vi "Intake Rotation Execute.vi"() -> ()   [LabVIEW 2017]
uses:
  Intake Rotation Control Type.ctl
  <vilib>/Rock Robotics/WPI/DriverStation/WPI_DriverStationRobotMode2.ctl
  Intake Rotation Notifier.ctl
  Arm Enum States.ctl
  <vilib>/Rock Robotics/WPI/ThirdParty/Phoenix-LabVIEW/Motor Controller/Controls/CTRE_Phoenix_MotorControl_ControlMode.ctl
  Intake Rotation Globals.vi
  Utility VIs/Refnum Names.vi
  Robot Global Data.vi
  Lift/Lift Globals.vi
panel:
  out "error out 3":errorcluster
  out "error out 2":errorcluster
  in  "Up kP Stow":dbl=0.001
  out "Maintain Position 2":i32
  in  "Min Output":dbl=-0.5
  in  "Max Ouput":dbl=0.6
  out "error out":errorcluster
  out "Maintain Position":i32
  in  "Lift Point":i32=6000
  in  "Kp Up":dbl=0.0003
  in  "Kp Down":dbl=0.0003
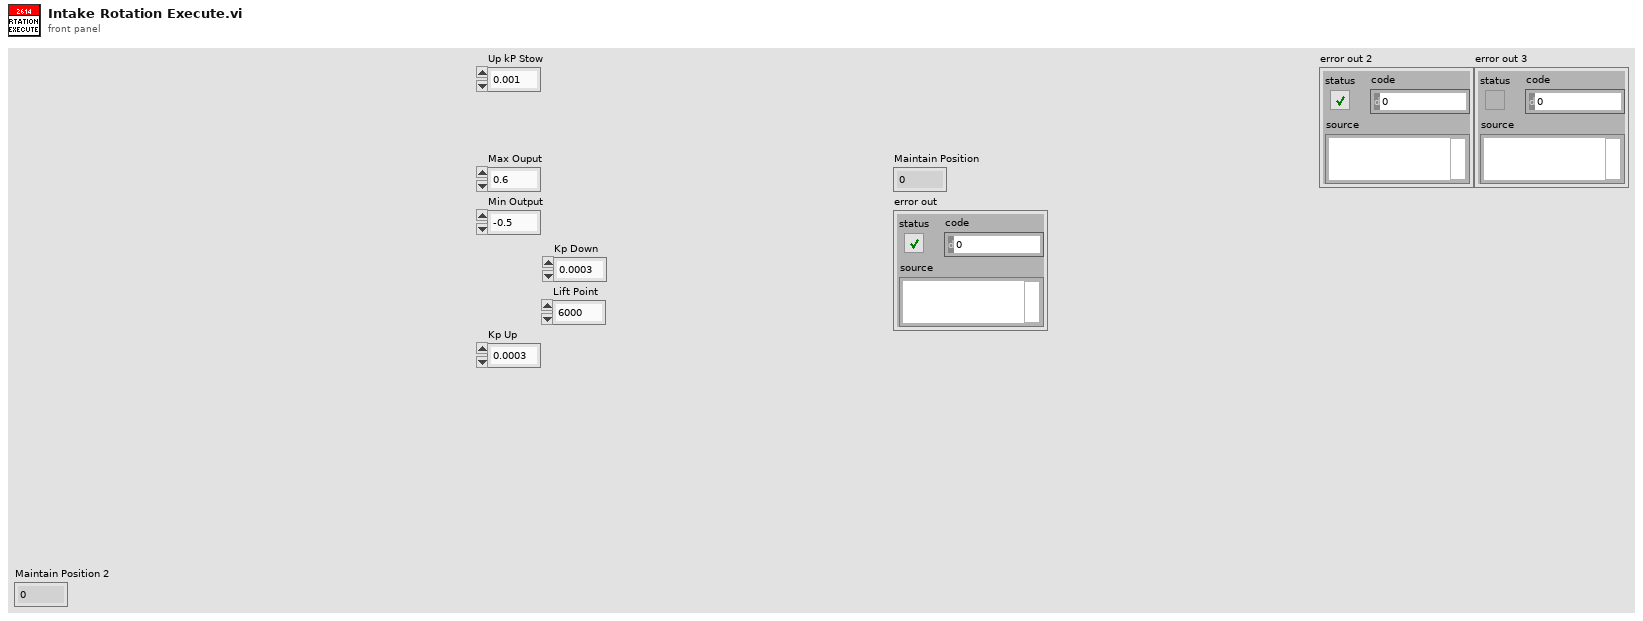
[diagram p1: front panel]
types:
  T1 = typedef "WPI_MotorControlDeviceRef.ctl" = cluster{"DeviceStatus":errorcluster, "Type":T2, "PWM":cluster{"PWM Channel":T3, "DeadBand":T4}, "CAN":cluster{"Device Number":u8, "SetOutput VI Ref":variant, "GetOutput VI Ref":variant, "Enable VI Ref":variant, "Disable VI Ref":variant, "Data":variant}, "Invert":bool, "DIO PWM":cluster{"PWM \"Enable\" Channel":T3, "DIOChannel":T5, "PWM Rate":dbl}}
  T2 = typedef "WPI_MotorControlType.ctl" = enum16{"PWM", "CAN", "DIO PWM"}
  T3 = typedef "FPGA_DIOPWMChannel.ctl" = enum8{"PWM 0", "PWM 1", "PWM 2", "PWM 3", "PWM 4", "PWM 5", "PWM 6", "PWM 7", "PWM 8", "PWM 9", "PWM MXP 0", "PWM MXP 1", "PWM MXP 2", "PWM MXP 3", "PWM MXP 4", "PWM MXP 5", "PWM MXP 6", "PWM MXP 7", "PWM MXP 8", "PWM MXP 9", "Invalid"}
  T4 = typedef "WPI_PWMDeadband.ctl" = cluster{"Name":string, "maxPositivePwm":i32, "minPositivePwm":i32, "centerPwm":i32, "maxNegativePwm":i32, "minNegativePwm":i32, "angularRange":u16}
  T5 = typedef "FPGA_DIOChannel.ctl" = enum8{"DIO 0", "DIO 1", "DIO 2", "DIO 3", "DIO 4", "DIO 5", "DIO 6", "DIO 7", "DIO 8", "DIO 9", "DIO MXP 0", "DIO MXP 1", "DIO MXP 2", "DIO MXP 3", "DIO MXP 4", "DIO MXP 5", "DIO MXP 6", "DIO MXP 7", "DIO MXP 8", "DIO MXP 9", "DIO MXP 10", "DIO MXP 11", "DIO MXP 12", "DIO MXP 13", "DIO MXP 14", "DIO MXP 15", "SPI Port CS1", "SPI Port CS2", "SPI Port CS3", "SPI Port MISO", "SPI Port MOSI", "Invalid"}
  T6 = typedef "Intake Rotation Control Type.ctl" = enum16{"No Op", "Manual Up", "Position", "Manual Down", "PositionAuto"}
  T7 = typedef "WPI_DriverStationRobotMode2.ctl" = enum16{"Autonomous Disabled", "Autonomous Enabled", "Teleop Disabled", "Teleop Enabled", "Disconnected", "Finish", "Test Disabled", "Test Enabled", "Emergency Stopped"}
  T8 = typedef "Intake Rotation Notifier.ctl" = cluster{"Step":i32, "Intake Rotation Control Type":T6, "Parameter 1":dbl, "Parameter 2":dbl, "Intake Rotation Notifier":refnum<notifier>, "Manual Up":bool, "Manual Down":bool, "Climb":bool, "Switch":bool, "Scale Low":bool, "Scale High":bool, "Stow":bool, "Load":bool, "Scale Mid":bool, "Exchange":bool, "Set Position":T9, "Portal":bool}
  T9 = typedef "Arm Enum States.ctl" = enum16{"Current Position", "Climb", "Load", "Portal", "Switch", "Scale High", "Scale Mid", "Scale Low", "Exchange", "Stow"}
  T10 = typedef "CTRE_Phoenix_MotorControl_ControlMode.ctl" = u16
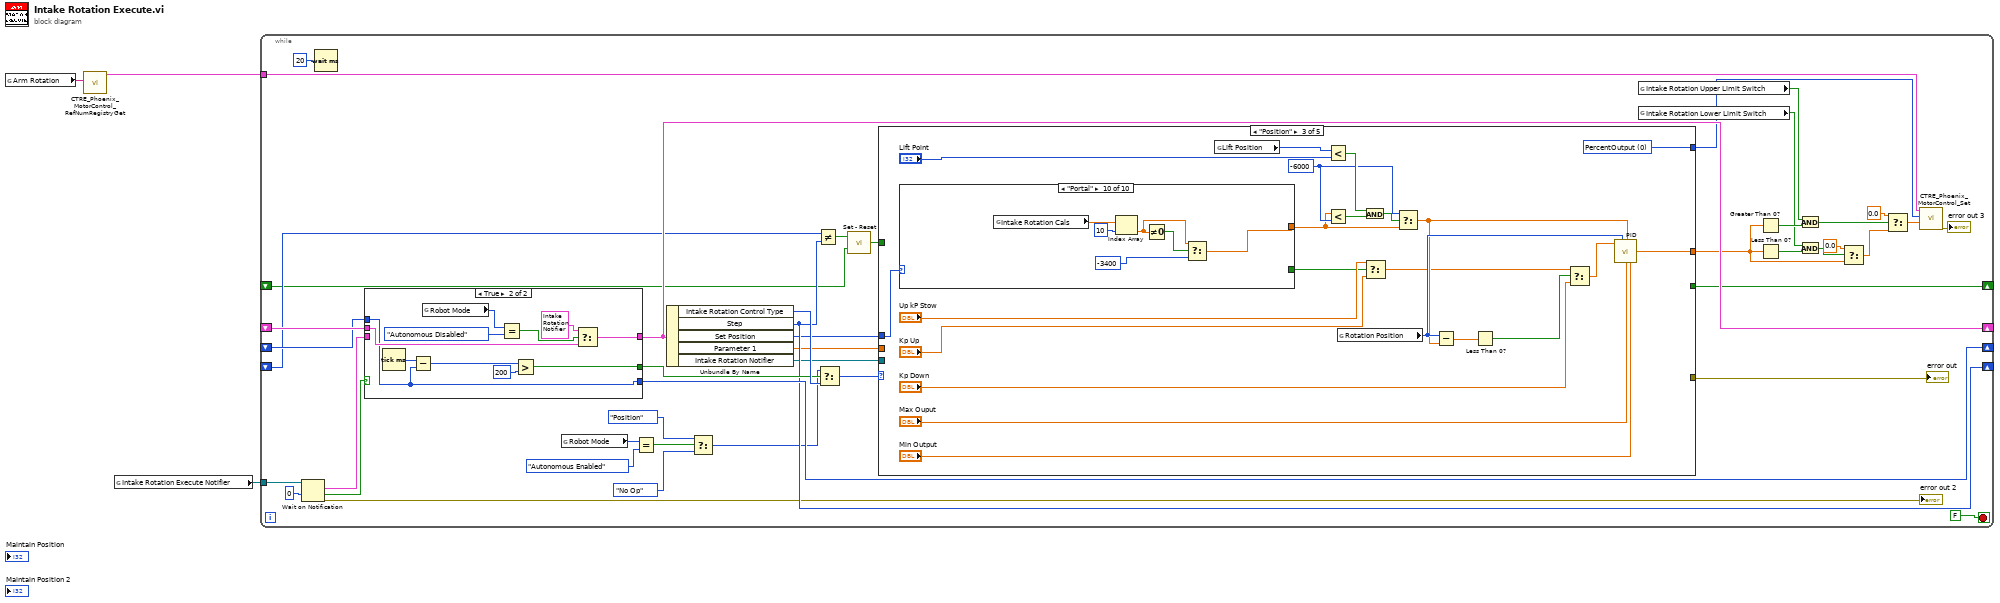
[diagram p0: block diagram]
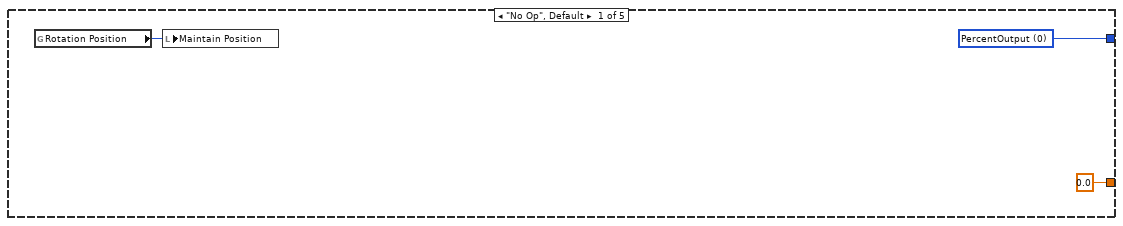
[diagram p2: hidden frame]
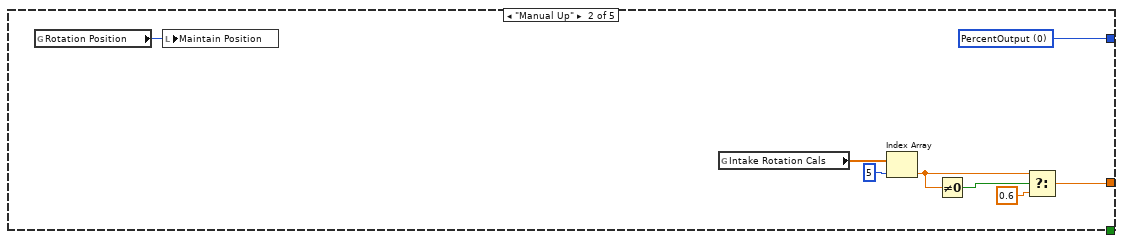
[diagram p3: hidden frame]
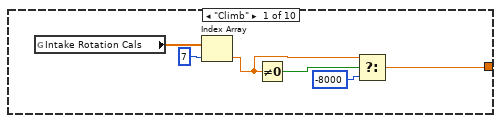
[diagram p4: hidden frame]
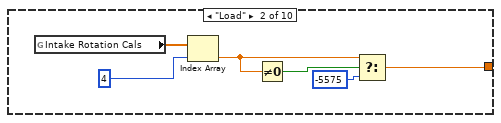
[diagram p5: hidden frame]
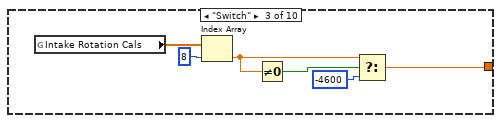
[diagram p6: hidden frame]
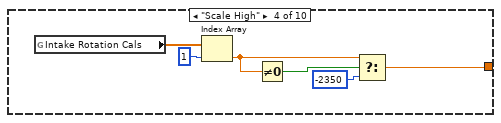
[diagram p7: hidden frame]
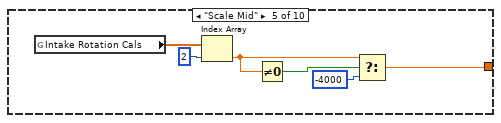
[diagram p8: hidden frame]
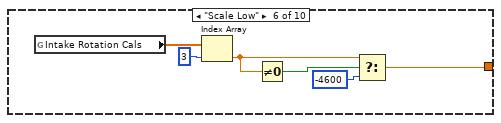
[diagram p9: hidden frame]
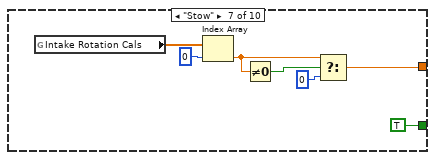
[diagram p10: hidden frame]
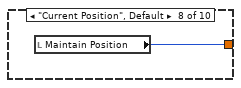
[diagram p11: hidden frame]
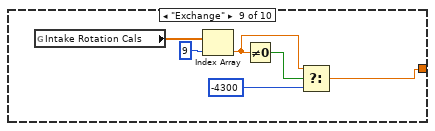
[diagram p12: hidden frame]
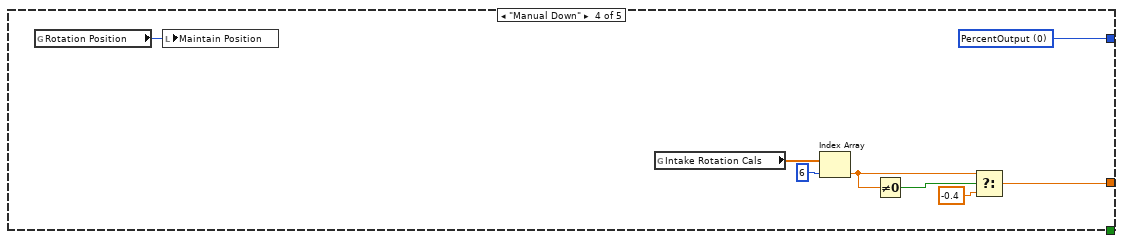
[diagram p13: hidden frame]
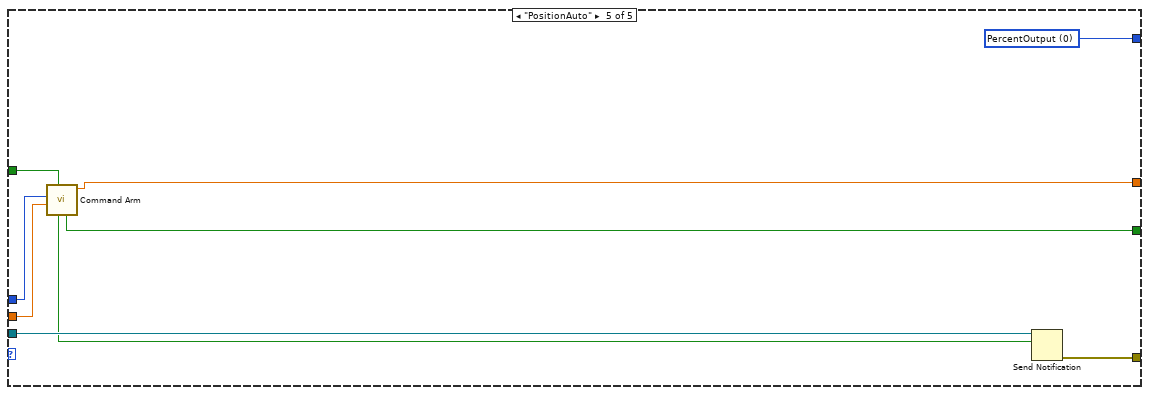
[diagram p14: hidden frame]
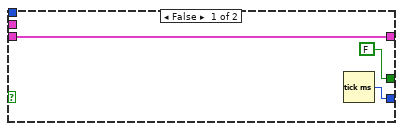
[diagram p15: hidden frame]
diagram:
  n1 = global read "Refnum Names.vi" "Arm Rotation"() -> (w2:string)
  n2 = call <vilib>:"CTRE_Phoenix_MotorControl_RefNumRegistryGet.vi"("refnum name"=w2) -> ("PhoenixMotorControlDevRef"=w1:T1)  [unwired: 9 in, 1 out]
  n3 = global read "Intake Rotation Globals.vi" "Intake Rotation Execute Notifier"() -> (w3:refnum<notifier>)
  n4 = while {
    tunnel: w3 -> [w45]
    shift-right: [w38] -> _
    shift-left: _ -> [w42]
    shift-right: [w40] -> _
    shift-left: _ -> [w39]
    shift-right: [w34] -> _
    shift-left: _ -> [w35]
    shift-right: [w31] -> _
    shift-left: _ -> [w30]
    tunnel: w1 -> [w29]
    stop <- FALSE stop-if-true
    n5 = Wait on Notification(notifier=w45, timeout in ms (-1)=0) -> (notification=w41:T8, timed out?=w43:bool, error out=→"error out 2":errorcluster)  [unwired: 2 in, 1 out]
    n6 = Wait (ms)(milliseconds to wait=u32 20) -> ()  [unwired: 1 out]
    n7 = case shown="True" w43 {
      tunnel: w42 -> [_ w166]
      tunnel: [w156 w165] -> w38
      tunnel: w41 -> [w156 _]
      tunnel: [w155 w158] -> w40
      tunnel: w39 -> [_ w158]
      tunnel: [FALSE w161] -> w36
      frame False {
        n8 = Tick Count (ms)() -> (millisecond timer value=w155:u32)
      }
      frame True {
        n9 = Tick Count (ms)() -> (millisecond timer value=w164:u32)
        n10 = Subtract(x=w164, y=w158) -> (x-y=w163:u32)
        n11 = global read "Robot Global Data.vi" "Robot Mode"() -> (w160:T7)
        n12 = Equal?(x=w160, y=WPI_DriverStationRobotMode2."Autonomous Disabled") -> (x = y?=w167:bool)
        n13 = Greater?(x=w163, y=u32 200) -> (0:w161:bool)
        n14 = Select(t=T8 {"Step"=0, "Intake Rotation Control Type"=enum."No Op", "Parameter 1"=0.0, "Parameter 2"=0.0, "Intake Rotation Notifier"=refnum, "Manual Up"=FALSE, "Manual Down"=FALSE, "Climb"=FALSE, "Switch"=FALSE, "Scale Low"=FALSE, "Scale High"=FALSE, "Stow"=FALSE, "Load"=FALSE, "Scale Mid"=FALSE, "Exchange"=FALSE, "Set Position"=enum."Current Position", "Portal"=FALSE} ("Intake Rotation Notifier"), s=w167, f=w166) -> (s? t:f=w165:T8)
      }
    }
    n15 = global read "Robot Global Data.vi" "Robot Mode"() -> (w13:T7)
    n16 = Equal?(x=w13, y=WPI_DriverStationRobotMode2."Autonomous Enabled") -> (x = y?=w12:bool)
    n17 = Unbundle By Name(w38) -> ("Intake Rotation Control Type"=w37:T6, "Step"=w34:i32, "Set Position"=w27:T9, "Parameter 1"=w7:dbl, "Intake Rotation Notifier"=w15:refnum<notifier>)
    n18 = Select(t=Intake_Rotation_Control_Type."Position", s=w12, f=Intake_Rotation_Control_Type."No Op" ("t")) -> (s? t:f=w8:T6)
    n19 = Not Equal?(x=w35, y=w34) -> (x != y?=w33:bool)
    n20 = Select(t=w8, s=w36, f=w37) -> (s? t:f=w10:T6)
    n21 = call "Set - Reset.vi"("Reset"=w30, "Set"=w33) -> ("Output"=w32:bool)
    n22 = case shown="\"Position\"" w10 {
      tunnel: w32 -> [_ _ _ _ w151]
      tunnel: [_ _ _ _ w149] -> w31
      tunnel: [w50 w58 w80 w144 w153] -> w28
      tunnel: [0.0 ("Output") w51 w63 w137 w150] -> w17
      tunnel: w27 -> [_ _ w65 _ w147]
      tunnel: w15 -> [_ _ _ _ w152]
      tunnel: w7 -> [_ _ _ _ w146]
      tunnel: [_ _ _ _ w145] -> w6
      frame "No Op", Default {
        w50 = T10 0 items=["PercentOutput"=0, "Position"=1, "Velocity"=2, "Current"=3, "Follower"=5, "MotionProfile"=6, "MotionMagic"=7, "MotionMagicArc"=8, "MotionProfileArc"=10, "Disabled"=15] ("Control Mode")
        n23 = global read "Intake Rotation Globals.vi" "Rotation Position"() -> (w48:i32)
        n24 = local write "Maintain Position"(w48) -> ()
      }
      frame "Manual Up" {
        w58 = T10 0 items=["PercentOutput"=0, "Position"=1, "Velocity"=2, "Current"=3, "Follower"=5, "MotionProfile"=6, "MotionMagic"=7, "MotionMagicArc"=8, "MotionProfileArc"=10, "Disabled"=15] ("Control Mode")
        n25 = global read "Intake Rotation Globals.vi" "Rotation Position"() -> (w57:i32)
        n26 = local write "Maintain Position"(w57) -> ()
        n27 = global read "Intake Rotation Globals.vi" "Intake Rotation Cals"() -> (w52:dbl[])
        n28 = Index Array(array=w52, index=5) -> (element=w55:dbl)
        n29 = Not Equal To 0?(x=w55) -> (x != 0?=w54:bool)
        n30 = Select(t=w55, s=w54, f=0.6) -> (s? t:f=w51:dbl)
      }
      frame "Position" {
        w70 = -6000 ("y")
        w80 = T10 0 items=["PercentOutput"=0, "Position"=1, "Velocity"=2, "Current"=3, "Follower"=5, "MotionProfile"=6, "MotionMagic"=7, "MotionMagicArc"=8, "MotionProfileArc"=10, "Disabled"=15] ("Control Mode")
        n31 = case shown="\"Portal\"" w65 {
          tunnel: [w82 w87 w93 w99 w105 w111 w118 w124 w127 w131] -> w64
          tunnel: [_ _ _ _ _ _ TRUE _ _ _] -> w59
          frame "Climb" {
            n32 = global read "Intake Rotation Globals.vi" "Intake Rotation Cals"() -> (w86:dbl[])
            n33 = Index Array(array=w86, index=7) -> (element=w81:dbl)
            n34 = Not Equal To 0?(x=w81) -> (x != 0?=w84:bool)
            n35 = Select(t=w81, s=w84, f=-8000) -> (s? t:f=w82:dbl)
          }
          frame "Load" {
            n36 = global read "Intake Rotation Globals.vi" "Intake Rotation Cals"() -> (w92:dbl[])
            n37 = Index Array(array=w92, index=4) -> (element=w88:dbl)
            n38 = Not Equal To 0?(x=w88) -> (x != 0?=w90:bool)
            n39 = Select(t=w88, s=w90, f=-5575) -> (s? t:f=w87:dbl)
          }
          frame "Switch" {
            n40 = global read "Intake Rotation Globals.vi" "Intake Rotation Cals"() -> (w98:dbl[])
            n41 = Index Array(array=w98, index=8) -> (element=w94:dbl)
            n42 = Not Equal To 0?(x=w94) -> (x != 0?=w96:bool)
            n43 = Select(t=w94, s=w96, f=-4600) -> (s? t:f=w93:dbl)
          }
          frame "Scale High" {
            n44 = global read "Intake Rotation Globals.vi" "Intake Rotation Cals"() -> (w104:dbl[])
            n45 = Index Array(array=w104, index=1) -> (element=w100:dbl)
            n46 = Not Equal To 0?(x=w100) -> (x != 0?=w102:bool)
            n47 = Select(t=w100, s=w102, f=-2350) -> (s? t:f=w99:dbl)
          }
          frame "Scale Mid" {
            n48 = global read "Intake Rotation Globals.vi" "Intake Rotation Cals"() -> (w110:dbl[])
            n49 = Index Array(array=w110, index=2) -> (element=w106:dbl)
            n50 = Not Equal To 0?(x=w106) -> (x != 0?=w108:bool)
            n51 = Select(t=w106, s=w108, f=-4000) -> (s? t:f=w105:dbl)
          }
          frame "Scale Low" {
            n52 = global read "Intake Rotation Globals.vi" "Intake Rotation Cals"() -> (w116:dbl[])
            n53 = Index Array(array=w116, index=3) -> (element=w112:dbl)
            n54 = Not Equal To 0?(x=w112) -> (x != 0?=w114:bool)
            n55 = Select(t=w112, s=w114, f=-4600) -> (s? t:f=w111:dbl)
          }
          frame "Stow" {
            n56 = global read "Intake Rotation Globals.vi" "Intake Rotation Cals"() -> (w123:dbl[])
            n57 = Index Array(array=w123, index=0) -> (element=w119:dbl)
            n58 = Not Equal To 0?(x=w119) -> (x != 0?=w121:bool)
            n59 = Select(t=w119, s=w121, f=0) -> (s? t:f=w118:dbl)
          }
          frame "Current Position", Default {
            n60 = local read "Maintain Position"() -> (w124:i32)
          }
          frame "Exchange" {
            n61 = global read "Intake Rotation Globals.vi" "Intake Rotation Cals"() -> (w130:dbl[])
            n62 = Index Array(array=w130, index=9) -> (element=w125:dbl)
            n63 = Not Equal To 0?(x=w125) -> (x != 0?=w128:bool)
            n64 = Select(t=w125, s=w128, f=-4300) -> (s? t:f=w127:dbl)
          }
          frame "Portal" {
            n65 = global read "Intake Rotation Globals.vi" "Intake Rotation Cals"() -> (w136:dbl[])
            n66 = Index Array(array=w136, index=10) -> (element=w133:dbl)
            n67 = Not Equal To 0?(x=w133) -> (x != 0?=w134:bool)
            n68 = Select(t=w133, s=w134, f=-3400) -> (s? t:f=w131:dbl)
          }
        }
        n69 = global read "Lift Globals.vi" "Lift Position"() -> (w75:i32)
        n70 = Less?(x=w75, y="Lift Point") -> (x < y?=w73:bool)
        n71 = Less?(x=w64, y=w70) -> (x < y?=w72:bool)
        n72 = global read "Intake Rotation Globals.vi" "Rotation Position"() -> (w69:i32)
        n73 = And(x=w73, y=w72) -> (x .and. y?=w71:bool)
        n74 = Select(t="Up kP Stow", s=w59, f="Kp Up") -> (s? t:f=w62:dbl)
        n75 = Select(t=w70, s=w71, f=w64) -> (s? t:f=w68:dbl)
        n76 = Subtract(x=w69, y=w68) -> (x-y=w79:dbl)
        n77 = Less Than 0?(x=w79) -> (x < 0?=w78:bool)
        n78 = Select(t=w62, s=w78, f="Kp Down") -> (s? t:f=w77:dbl)
        n79 = call "PID.vi"("Kp"=w77, "Process Variable"=w69, "Goal"=w68, "Max Ouput"="Max Ouput", "Min Output"="Min Output") -> ("Command"=w63:dbl)  [unwired: 8 in, 2 out]
      }
      frame "Manual Down" {
        w144 = T10 0 items=["PercentOutput"=0, "Position"=1, "Velocity"=2, "Current"=3, "Follower"=5, "MotionProfile"=6, "MotionMagic"=7, "MotionMagicArc"=8, "MotionProfileArc"=10, "Disabled"=15] ("Control Mode")
        n80 = global read "Intake Rotation Globals.vi" "Rotation Position"() -> (w143:i32)
        n81 = local write "Maintain Position"(w143) -> ()
        n82 = global read "Intake Rotation Globals.vi" "Intake Rotation Cals"() -> (w142:dbl[])
        n83 = Index Array(array=w142, index=6) -> (element=w139:dbl)
        n84 = Not Equal To 0?(x=w139) -> (x != 0?=w140:bool)
        n85 = Select(t=w139, s=w140, f=-0.4) -> (s? t:f=w137:dbl)
      }
      frame "PositionAuto" {
        w153 = T10 0 items=["PercentOutput"=0, "Position"=1, "Velocity"=2, "Current"=3, "Follower"=5, "MotionProfile"=6, "MotionMagic"=7, "MotionMagicArc"=8, "MotionProfileArc"=10, "Disabled"=15] ("Control Mode")
        n86 = call "Command Arm.vi"("Startup"=w151, "Timeout"=w146, "Set Position"=w147) -> ("Arm Out"=w150:dbl, "Reinit"=w149:bool, "Completed"=w148:bool)  [unwired: 6 in]
        n87 = Send Notification(notification=w148, notifier=w152) -> (error out=w145:errorcluster)  [unwired: 1 in, 1 out]
      }
    }
    "error out" <- w6
    n88 = global read "Intake Rotation Globals.vi" "Intake Rotation Upper Limit Switch"() -> (w24:bool)
    n89 = global read "Intake Rotation Globals.vi" "Intake Rotation Lower Limit Switch"() -> (w19:bool)
    n90 = Greater Than 0?(x=w17) -> (x > 0?=w23:bool)
    n91 = Less Than 0?(x=w17) -> (x < 0?=w18:bool)
    n92 = And(x=w24, y=w23) -> (x .and. y?=w22:bool)
    n93 = And(x=w19, y=w18) -> (x .and. y?=w20:bool)
    n94 = Select(t=0.0, s=w20, f=w17) -> (s? t:f=w26:dbl)
    n95 = Select(t=0.0, s=w22, f=w26) -> (s? t:f=w25:dbl)
    n96 = call <vilib>:"CTRE_Phoenix_MotorControl_Set.vi"("Output"=w25, "Control Mode"=w28, "PhoenixMotorControlDevRef"=w29) -> ("error out"=→"error out 3":errorcluster)  [unwired: 7 in, 1 out]
  }
